vi "Eurotherm 32xx Series Process Value Monitoring.vi"() -> ()   [LabVIEW 2010]
doc: "This example demonstrates process value monitoring only.\n\nNote:\nEnter correct VISA Resource Descriptor, Device Address and Baud Rate into front-panel controls before you run this VI!\nBefore start this VI must be controller configuration ready and controller must run."
uses:
  <instrlib>/Eurotherm 32xx Series/Eurotherm 32xx Series.lvlib
panel:
  in  "Serial Configuration":T1={"Baud Rate (19200)"=19200, "Parity (0: None)"=0, "Break Length (0)"=20} {"Break Length (0)" items=["0"=10, "1.5"=15, "2.0"=20]; "Parity (0: None)" items=["None", "Odd", "Even"]; "Baud Rate (19200)" items=["1200"=1200, "2400"=2400, "4800"=4800, "9600"=9600, "19200"=19200]}
  in  "stop":bool
  out "Process Value - Chart":sgl(graph)
  out "Process Value":sgl
  in  "Unit Address (1)":u8=1 min=1 max=254
  in  "VISA resource name":refnum<visa-resource-name>
  in  "Acknowledge All Alarms":bool
  out "New ALARM !":bool
  # "(c) 2010 <Invensys Eurotherm>.  ALL RIGHTS RESERVED."
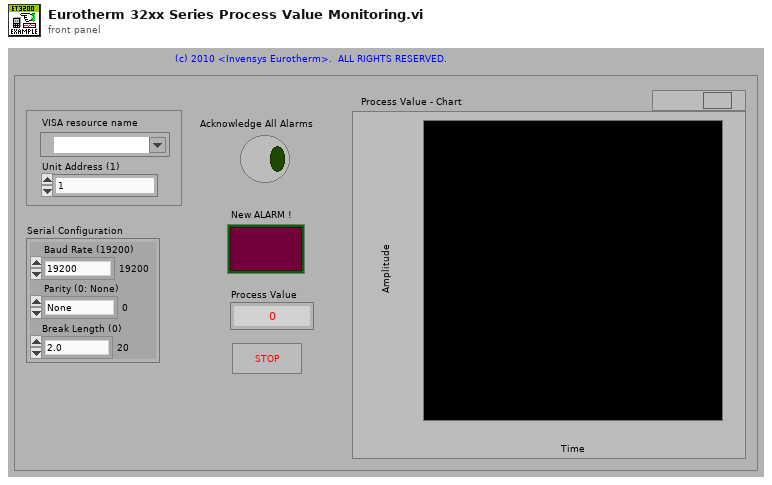
[diagram p1: front panel]
types:
  T1 = cluster{"Baud Rate (19200)":u32, "Parity (0: None)":u16, "Break Length (0)":u16}
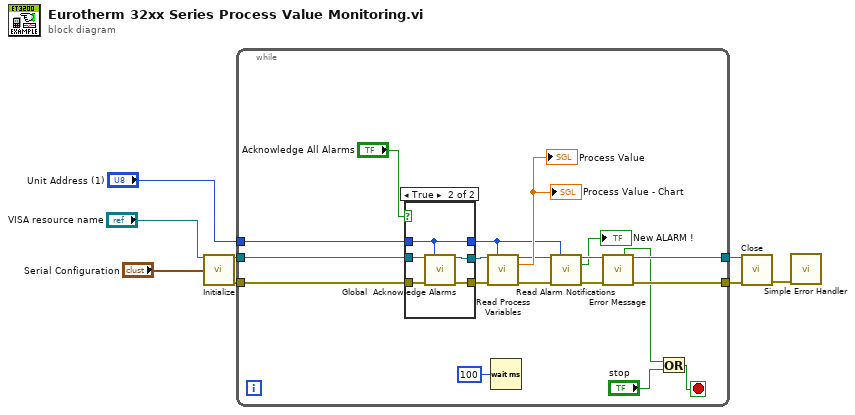
[diagram p0: block diagram]
diagram:
  n1 = call <instrlib>:"Initialize.vi"("VISA resource name"="VISA resource name", "Serial Configuration"="Serial Configuration") -> ("VISA resource name out"=w4:refnum<visa-resource-name>, "error out"=w3:errorcluster)  [unwired: 12 in]
  n2 = while {
    tunnel: w4 -> [w10]
    tunnel: w3 -> [w9]
    tunnel: "Unit Address (1)" -> [w11]
    tunnel: [w25] -> w6
    tunnel: [w24] -> w7
    stop <- w21 stop-if-true
    n3 = case shown="True" "Acknowledge All Alarms" {
      tunnel: w10 -> [w29 w35]
      tunnel: w9 -> [w28 w34]
      tunnel: [w29 w33] -> w13
      tunnel: [w28 w32] -> w12
      tunnel: w11 -> [w30 w31]
      tunnel: [w30 w31] -> w14
      frame False {
      }
      frame True {
        n4 = call <instrlib>:"Global  Acknowledge Alarms.vi"("VISA resource name"=w35, "Unit Address (1)"=w31, "error in (no error)"=w34) -> ("VISA resource name out"=w33:refnum<visa-resource-name>, "error out"=w32:errorcluster)  [unwired: 11 in]
      }
    }
    n5 = call <instrlib>:"Read Process Variables.vi"("VISA resource name"=w13, "Unit Address (1)"=w14, "error in (no error)"=w12) -> ("VISA resource name out"=w16:refnum<visa-resource-name>, "Process Value"=→"Process Value" →"Process Value - Chart":sgl, "error out"=w15:errorcluster)  [unwired: 9 in, 1 out]
    n6 = Wait (ms)(milliseconds to wait=u32 100) -> ()  [unwired: 1 out]
    n7 = call <instrlib>:"Read Alarm Notifications.vi"("VISA resource name"=w16, "Unit Address (1)"=w14, "error in (no error)"=w15) -> ("VISA resource name out"=w27:refnum<visa-resource-name>, "New Alarm"=→"New ALARM !":bool, "error out"=w26:errorcluster)  [unwired: 10 in]
    n8 = call <instrlib>:"Error Message.vi"("VISA resource name"=w27, "error in (no error)"=w26) -> ("Status"=w19:bool, "VISA resource name out"=w25:refnum<visa-resource-name>, "error out"=w24:errorcluster)  [unwired: 9 in, 2 out]
    n9 = Or(x=w19, y="stop") -> (x .or. y?=w21:bool)
  }
  n10 = call <instrlib>:"Close.vi"("VISA resource name"=w6, "error in (no error)"=w7) -> ("error out"=w2:errorcluster)  [unwired: 13 in]
  n11 = call <vilib>:"Simple Error Handler.vi"("error in (no error)"=w2) -> ()  [unwired: 4 in, 5 out]
